vi "Editor Soglie pedrollo.vi"(11 "COLLEGAMENTO":u16(ring) items=["3-MOTORE C.A."]) -> ()   [LabVIEW 2019]
uses:
  TypeDef/DT TRASFORMATORE.ctl
  TypeDef/DT POMPA EXX.ctl
  TypeDef/DT POMPA.ctl
  TypeDef/DT MOTORE CC.ctl
  TypeDef/MOTORE EEX.ctl
  TypeDef/DT MOTORE CA.ctl
  TypeDef/DT GENERICO.ctl
  TypeDef/DT GENERATORE.ctl
  <vilib>/Utility/file.llb/Read Delimited Spreadsheet (string).vi
  <vilib>/Utility/file.llb/Write Delimited Spreadsheet (string).vi
panel:
  in  "Tab dati macchina":T1(tab)=enum."Page 4"
  in  "DATI MACCHINA-GENERATORE":T2
  in  "DATI MACCHINA-GENERICO":T3
  in  "DATI MACCHINA-MOTORE C.A.":T4
  in  "DATI MACCHINA-MOTORE EEX":T5
  in  "DATI MACCHINA-MOTORE C.C.":T6
  in  "DATI MACCHINA-POMPA":T7
  in  "DATI MACCHINA-POMPA EEX":T8
  in  "DATI MACCHINA-TRASFORMATORE":T9
  in  "salva soglie":bool
  in  "elimina soglia":bool
  in  "stop":bool
  in  "Cluster % NOMINALE":T10 {"VALORE NOMINALE BOLLETTINO" items=["3-MOTORE C.A.>>MARCA", "3-MOTORE C.A.>>TIPO", "3-MOTORE C.A.>>MATRICOLA", "3-MOTORE C.A.>>N°POLI", "3-MOTORE C.A.>>POTENZA [kW]", "3-MOTORE C.A.>>TENSIONE [V]", "3-MOTORE C.A.>>CORRENTE [A]", "3-MOTORE C.A.>>FREQUENZA [Hz]", "3-MOTORE C.A.>>RPM NOMINALI", "3-MOTORE C.A.>>RPM MAX", "3-MOTORE C.A.>>COSTRUTTORE", "3-MOTORE C.A.>>MODELLO Nr.", "3-MOTORE C.A.>>TIPO SERVIZIO", "3-MOTORE C.A.>>DESIGN", "3-MOTORE C.A.>>CLASSE ISOL", "3-MOTORE C.A.>>STATORE", "3-MOTORE C.A.>>ROTORE", "3-MOTORE C.A.>>NOTE"]; "RITARDO INTERVENTO" format="%#_g s"; "SOGLIA SUPERIORE" format="%#_g %"; "SOGLIA INFERIORE" format="%#_g %"}
  in  "SOGLIE INSERITE":i32(listbox)
  in  "Cluster COSTANTE":T11
  in  "costante \\ dinamica":bool=TRUE caption="SOGLIA COSTANTE\n\nSOGLIA DINAMICA\n% VALORE NOMINALE"
  in  "inserisci soglia":bool
  in  "Listbox":i32(listbox)
  # "GESTIONE SOGLIE"
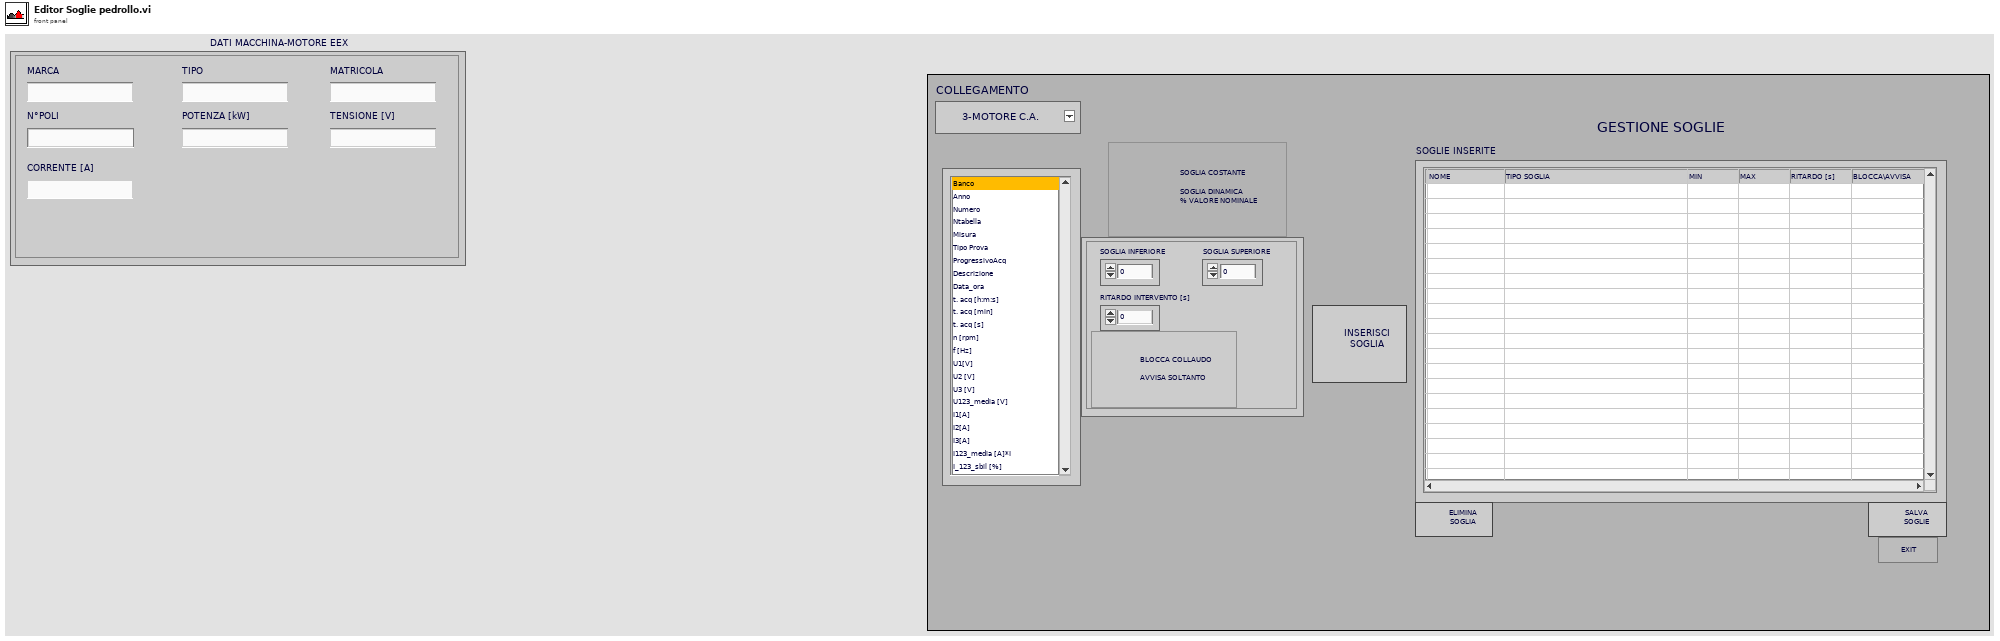
[diagram p1: front panel]
types:
  T1 = enum32{"Page 1", "Page 2", "Page 3", "Page 4", "Page 5", "Page 6", "Page 7", "Page 8"}
  T2 = typedef "DT GENERATORE.ctl" = cluster{"MARCA GENERATORE":string, "MARCA MOTORE":string, "MARCA ALTERNATORE":string, "MATRICOLA ALTERNATORE":string, "POTENZA [KVA]":string, "TENSIONE [V]":string, "CORRENTE [A]":string, "N° POLI":string, "GIRI [RPM]":string, "FREQUENZA [Hz]":string, "TENSIONE ECCIT.[V]":string, "CORRENTE ECCIT.[A]":string}
  T3 = typedef "DT GENERICO.ctl" = cluster{"MARCA":string, "TIPO":string, "MATRICOLA":string, "POTENZA [kW]":string, "TENSIONE [V]":string, "CORRENTE [A]":string}
  T4 = typedef "DT MOTORE CA.ctl" = cluster{"MARCA":string, "TIPO":string, "MATRICOLA":string, "N°POLI":string, "POTENZA [kW]":string, "TENSIONE [V]":string, "CORRENTE [A]":string, "FREQUENZA [Hz]":string, "RPM NOMINALI":string, "RPM MAX":string, "COSTRUTTORE":string, "MODELLO Nr.":string, "TIPO SERVIZIO":string, "DESIGN":string, "CLASSE ISOL":string, "STATORE":string, "ROTORE":string, "NOTE":string}
  T5 = typedef "MOTORE EEX.ctl" = cluster{"MARCA":string, "TIPO":string, "MATRICOLA":string, "N°POLI":string, "POTENZA [kW]":string, "TENSIONE [V]":string, "CORRENTE [A]":string}
  T6 = typedef "DT MOTORE CC.ctl" = cluster{"MARCA":string, "TIPO":string, "MATRICOLA":string, "POTENZA [kW]":string, "TENSIONE ARMAT.[V]":string, "CORRENTE ARMAT.[A]":string, "TENSIONE CAMPO [V]":string, "CORRENTE CAMPO [A]":string, "GIRI [RPM]":string, "TENSIONE DINAMO [V]":string}
  T7 = typedef "DT POMPA.ctl" = cluster{"MARCA":string, "TIPO":string, "MATRICOLA":string, "N°POLI":string, "POTENZA [kW]":string, "TENSIONE [V]":string, "CORRENTE [A]":string}
  T8 = typedef "DT POMPA EXX.ctl" = cluster{"MARCA":string, "TIPO":string, "MATRICOLA":string, "N°POLI":string, "POTENZA [kW]":string, "TENSIONE [V]":string, "CORRENTE [A]":string}
  T9 = typedef "DT TRASFORMATORE.ctl" = cluster{"MARCA":string, "TIPO":string, "MATRICOLA":string, "POTENZA [kW]":string, "TENSIONE PRIM. [V]":string, "CORRENTE PRIM. [A]":string, "TENSIONE SECON. [V]":string, "CORRENTE SECON. [A]":string, "GRUPPO CEI":string, "VCC%":string}
  T10 = cluster{"SOGLIA INFERIORE":dbl, "SOGLIA SUPERIORE":dbl, "RITARDO INTERVENTO":dbl, "blocca \\ avvisa":bool, "VALORE NOMINALE BOLLETTINO":u16}
  T11 = cluster{"SOGLIA INFERIORE":dbl, "SOGLIA SUPERIORE":dbl, "RITARDO INTERVENTO [s]":dbl, "blocca \\ avvisa":bool}
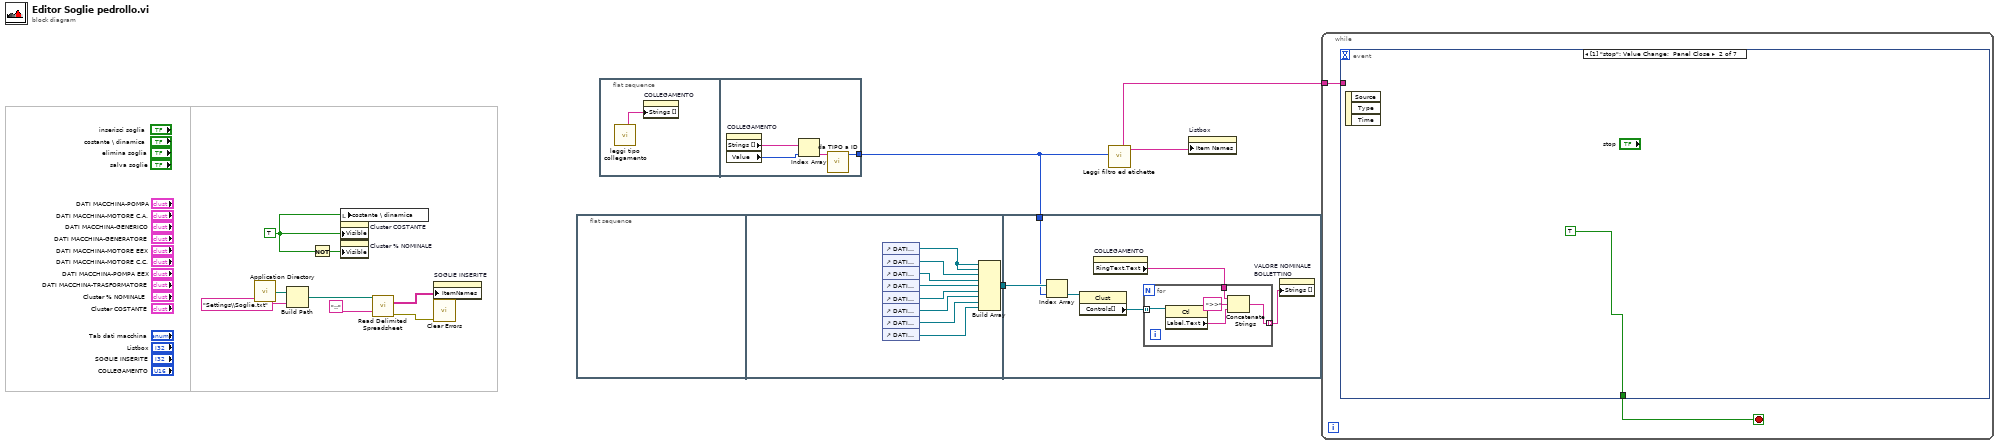
[diagram p0: block diagram]
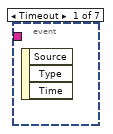
[diagram p2: hidden frame]
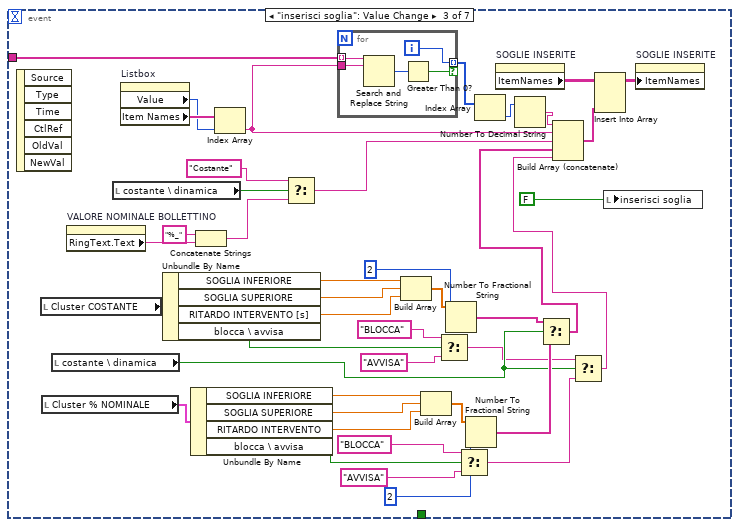
[diagram p3: hidden frame]
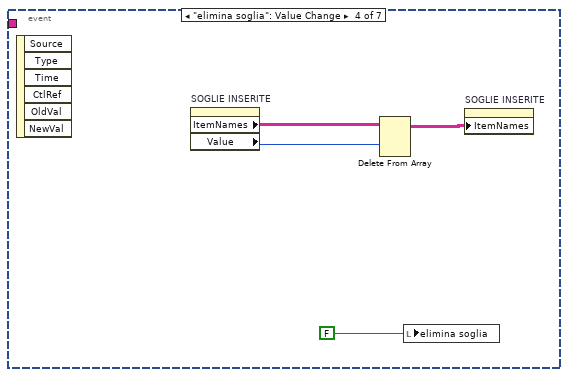
[diagram p4: hidden frame]
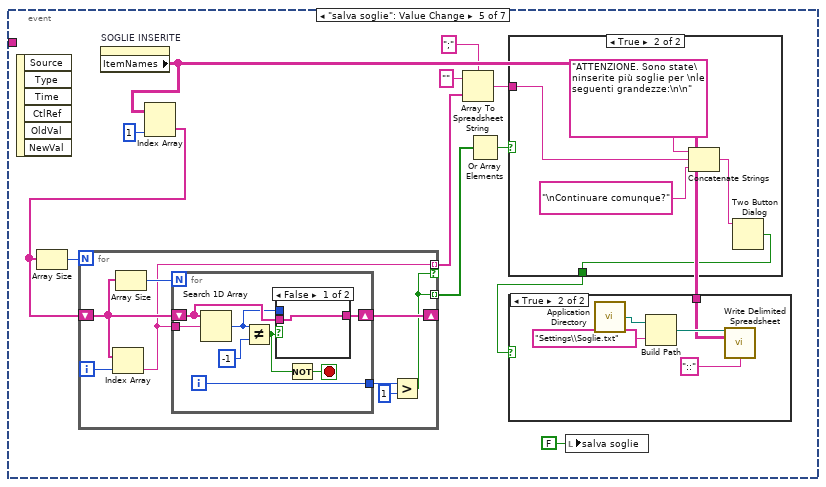
[diagram p5: hidden frame]
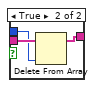
[diagram p6: hidden frame]
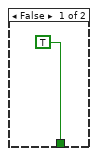
[diagram p8: hidden frame]
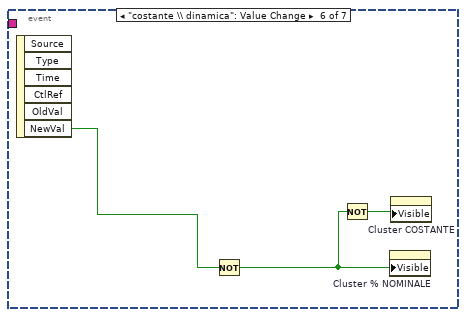
[diagram p9: hidden frame]
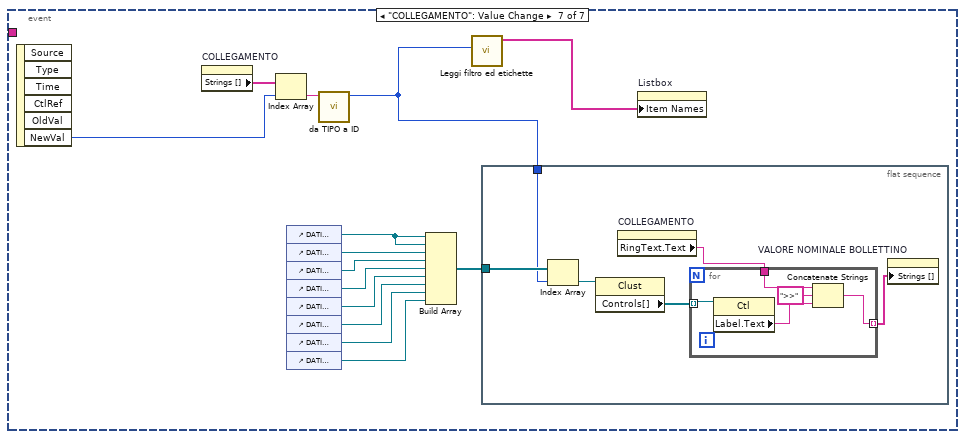
[diagram p10: hidden frame]
diagram:
  w6 = TRUE ("costante \\ dinamica")
  n1 = call <vilib>:"Application Directory.vi"() -> ("Application Directory"=w11:path)
  n2 = Build Path(base path=w11, name or relative path="Settings\\Soglie.txt") -> (appended path=w12:path)
  n3 = Not(x=w6) -> (.not. x?=w5:bool)
  n4 = local write "costante \\ dinamica"(w6) -> ()
  n5 = property on="Cluster COSTANTE" class="Clust (strict)"("Visible"=w6) -> ()  [unwired: 2 in, 2 out]
  n6 = property on="Cluster % NOMINALE" class="Clust (strict)"("Visible"=w5) -> ()  [unwired: 2 in, 2 out]
  n7 = call-poly <vilib>:"Read Delimited Spreadsheet.vi"("file path (dialog if empty)"=w12, "delimiter (\\t)"="::" ("delimiter (\\t)")) -> ("all rows"=w8:string[][], "error out"=w7:errorcluster)  [unwired: 8 in, 4 out]
  n8 = property on="SOGLIE INSERITE" class="MCListbox (strict)"("ItemNames"=w8) -> ()  [unwired: 2 in, 2 out]
  n9 = call <vilib>:"Clear Errors.vi"("error in (no error)"=w7) -> ()  [unwired: 5 in, 2 out]
  n10 = flat-sequence {
    tunnel: [w13] -> w1
    tunnel: w2 -> [w24]
    tunnel: w1 -> [w25]
    frame #0 {
    }
    frame #1 {
      n11 = control-ref of="DATI MACCHINA-GENERATORE"() -> (w14:refnum<vi>)
      n12 = control-ref of="DATI MACCHINA-GENERICO"() -> (w15:refnum<vi>)
      n13 = control-ref of="DATI MACCHINA-MOTORE C.A."() -> (w16:refnum<vi>)
      n14 = control-ref of="DATI MACCHINA-MOTORE EEX"() -> (w17:refnum<vi>)
      n15 = control-ref of="DATI MACCHINA-MOTORE C.C."() -> (w18:refnum<vi>)
      n16 = control-ref of="DATI MACCHINA-POMPA"() -> (w19:refnum<vi>)
      n17 = control-ref of="DATI MACCHINA-TRASFORMATORE"() -> (w20:refnum<vi>)
      n18 = control-ref of="DATI MACCHINA-POMPA EEX"() -> (w21:refnum<vi>)
      n19 = Build Array(w14, w14, w15, w16, w17, w18, w19, w20, w21) -> (w13:refnum<vi>[])
    }
    frame #2 {
      n20 = Index Array(array=w25, index=w24) -> (element=w23:refnum<vi>)
      n21 = property class="Clust"(reference=w23) -> ("Controls[]"=w26:refnum<vi>[])  [unwired: 1 in, 2 out]
      n22 = property on="COLLEGAMENTO" class="Ring (strict)"() -> ("RingText.Text"=w22:string)  [unwired: 2 in, 2 out]
      n23 = for {
        tunnel: w26 -> [w32] mode=indexing
        tunnel: [w30] -> w27 mode=indexing
        tunnel: w22 -> [w29]
        n24 = property class="Ctl"(reference=w32) -> ("Label.Text"=w31:string)  [unwired: 1 in, 2 out]
        n25 = Concatenate Strings(w29, ">>" ("string"), w31) -> (w30:string)
      }
      n26 = property on="VALORE NOMINALE BOLLETTINO" class="Ring (strict)"("Strings []"=w27) -> ()  [unwired: 2 in, 2 out]
    }
  }
  n27 = flat-sequence {
    tunnel: [w34] -> w2
    frame #0 {
      n28 = call "leggi tipo collegamento.vi"() -> ("lista"=w33:string[])  [unwired: 6 in, 5 out]
      n29 = property on="COLLEGAMENTO" class="Ring (strict)"("Strings []"=w33) -> ()  [unwired: 2 in, 2 out]
    }
    frame #1 {
      n30 = property on="COLLEGAMENTO" class="Ring (strict)"() -> ("Strings []"=w37:string[], "Value"=w36:u16)  [unwired: 2 in, 2 out]
      n31 = Index Array(array=w37, index=w36) -> (element=w35:string)
      n32 = call "da TIPO a ID.vi"("TIPO"=w35) -> ("ID"=w34:i32)  [unwired: 10 in]
    }
  }
  n33 = call "Leggi filtro ed etichette.vi"("ID COLLEGAMENTO"=w2) -> ("ETICHETTE"=w3:string[], "ALL"=w4:string[])  [unwired: 5 in, 4 out]
  n34 = property on="Listbox" class="LstBox (strict)"("Item Names"=w3) -> ()  [unwired: 2 in, 2 out]
  n35 = while {
    tunnel: w4 -> [w38]
    stop <- w39 stop-if-true
    n36 = event shown="[1] \"stop\": Value Change;  Panel Close" {
      selector: _ -> [_ _ _ _ _ _ _]
      dyn-events: _ -> [_ _ _ _ _ _ _]
      timeout: _ -> [_ _ _ _ _ _ _]
      tunnel: [_ TRUE _ _ _ _ _] -> w39
      tunnel: w38 -> [_ _ w47 _ _ _ _]
      event Timeout {
        n37 = event-data() -> ()  [unwired: 1 in, 3 out]
      }
      event "stop": Value Change; Panel Close {
        n38 = event-data() -> ()  [unwired: 1 in, 3 out]
      }
      event "inserisci soglia": Value Change {
        n39 = event-data() -> ()  [unwired: 1 in, 6 out]
        n40 = local read "Cluster COSTANTE"() -> (w68:T11)
        n41 = local read "Cluster % NOMINALE"() -> (w60:T10)
        n42 = local read "costante \\ dinamica"() -> (w56:bool)
        n43 = property on="VALORE NOMINALE BOLLETTINO" class="Ring (strict)"() -> ("RingText.Text"=w78:string)  [unwired: 2 in, 2 out]
        n44 = local read "costante \\ dinamica"() -> (w80:bool)
        n45 = property on="Listbox" class="LstBox (strict)"() -> ("Value"=w81:i32, "Item Names"=w82:string[])  [unwired: 2 in, 2 out]
        n46 = Unbundle By Name(w68) -> ("SOGLIA INFERIORE"=w72:dbl, "SOGLIA SUPERIORE"=w71:dbl, "RITARDO INTERVENTO [s]"=w70:dbl, "blocca \\ avvisa"=w75:bool)
        n47 = Unbundle By Name(w60) -> ("SOGLIA INFERIORE"=w64:dbl, "SOGLIA SUPERIORE"=w65:dbl, "RITARDO INTERVENTO"=w66:dbl, "blocca \\ avvisa"=w61:bool)
        n48 = Concatenate Strings("%_" ("string"), w78) -> (w76:string)
        n49 = Index Array(array=w82, index=w81) -> (element=w46:string)
        n50 = Select(t="Costante", s=w80, f=w76) -> (s? t:f=w41:string)
        n51 = for {
          tunnel: w47 -> [w87] mode=indexing
          tunnel: w46 -> [w86]
          tunnel: [w85] -> w45 mode=indexing if=w83
          i -> [w85]
          n52 = Search and Replace String(input string=w87, search string=w86) -> (number of replacements=w84:i32)  [unwired: 6 in, 3 out]
          n53 = Greater Than 0?(x=w84) -> (x > 0?=w83:bool)
        }
        n54 = Build Array(w72, w71, w70) -> (w69:dbl[])
        n55 = Build Array(w64, w65, w66) -> (w67:dbl[])
        n56 = Select(t="BLOCCA", s=w75, f="AVVISA") -> (s? t:f=w55:string)
        n57 = Number To Fractional String(number=w69, precision (6)=i16 2) -> (F-format string=w59:string[])  [unwired: 2 in]
        n58 = Select(t="BLOCCA", s=w61, f="AVVISA") -> (s? t:f=w54:string)
        n59 = Number To Fractional String(number=w67, precision (6)=i16 2) -> (F-format string=w58:string[])  [unwired: 2 in]
        n60 = Index Array(array=w45) -> (element=w44:i32)  [unwired: 1 in]
        n61 = property on="SOGLIE INSERITE" class="MCListbox (strict)"() -> ("ItemNames"=w52:string[][])  [unwired: 2 in, 2 out]
        n62 = Number To Decimal String(number=w44) -> (decimal integer string=w43:string)  [unwired: 1 in]
        n63 = Select(t=w59, s=w56, f=w58) -> (s? t:f=w57:string[])
        n64 = Select(t=w55, s=w56, f=w54) -> (s? t:f=w53:string)
        n65 = Build Array (concatenate)(w43, w46, w41, w57, w53) -> (w50:string[])
        n66 = Insert Into Array(array=w52, new element=w50) -> (w51:string[][])  [unwired: 2 in]
        n67 = local write "inserisci soglia"(FALSE ("inserisci soglia")) -> ()
        n68 = property on="SOGLIE INSERITE" class="MCListbox (strict)"("ItemNames"=w51) -> ()  [unwired: 2 in, 2 out]
      }
      event "elimina soglia": Value Change {
        n69 = event-data() -> ()  [unwired: 1 in, 6 out]
        n70 = property on="SOGLIE INSERITE" class="MCListbox (strict)"() -> ("ItemNames"=w91:string[][], "Value"=w90:i32)  [unwired: 2 in, 2 out]
        n71 = Delete From Array(array=w91, index (row)=w90) -> (array with subset deleted=w89:string[][])  [unwired: 2 in, 1 out]
        n72 = local write "elimina soglia"(FALSE ("elimina soglia")) -> ()
        n73 = property on="SOGLIE INSERITE" class="MCListbox (strict)"("ItemNames"=w89) -> ()  [unwired: 2 in, 2 out]
      }
      event "salva soglie": Value Change {
        n74 = event-data() -> ()  [unwired: 1 in, 6 out]
        n75 = property on="SOGLIE INSERITE" class="MCListbox (strict)"() -> ("ItemNames"=w102:string[][])  [unwired: 2 in, 2 out]
        n76 = Index Array(array=w102, index (col)=1 ("disabled index (col)")) -> (element=w94:string[])  [unwired: 1 in]
        n77 = Array Size(array=w94) -> (size(s)=w95:i32)
        n78 = for {
          N: w95 -> [_]
          tunnel: [w108] -> w93 mode=indexing if=w104
          shift-right: [w107] -> _
          shift-left: w94 -> [w110]
          tunnel: [w104] -> w92 mode=indexing
          i -> [w109]
          n79 = Index Array(array=w110, index=w109) -> (element=w108:string)
          n80 = Array Size(array=w110) -> (size(s)=w111:i32)
          n81 = for {
            N: w111 -> [_]
            tunnel: w108 -> [w119]
            shift-right: [w116] -> w107
            shift-left: w110 -> [w117]
            tunnel: [w112] -> w106
            i -> [w112]
            stop <- w113 stop-if-true
            n82 = Search 1D Array(1D array=w117, element=w119) -> (index of element=w115:i32)  [unwired: 1 in]
            n83 = Not Equal?(x=w115, y=-1) -> (x != y?=w114:bool)
            n84 = case shown="False" w114 {
              tunnel: w117 -> [w120 w123]
              tunnel: [w120 w122] -> w116
              tunnel: w115 -> [_ w121]
              frame False {
              }
              frame True {
                n85 = Delete From Array(array=w123, index=w121) -> (array with subset deleted=w122:string[])  [unwired: 1 in, 1 out]
              }
            }
            n86 = Not(x=w114) -> (.not. x?=w113:bool)
          }
          n87 = Greater?(x=w106, y=1) -> (0:w104:bool)
        }
        n88 = Array To Spreadsheet String(delimiter (Tab)=";", array=w93, 3:"" ("format string")) -> (spreadsheet string=w96:string)
        n89 = Or Array Elements(Boolean array=w92) -> (logical OR=w98:bool)
        n90 = case shown="True" w98 {
          tunnel: [TRUE w134] -> w97
          tunnel: w96 -> [_ w132]
          frame False {
          }
          frame True {
            n91 = Concatenate Strings("ATTENZIONE. Sono state\ninserite più soglie per \nle seguenti grandezze:\n\n" ("message"), w132, "\nContinuare comunque?" ("string")) -> (w131:string)
            n92 = Two Button Dialog(message=w131) -> (T button?=w134:bool)  [unwired: 2 in]
          }
        }
        n93 = case shown="True" w97 {
          tunnel: w102 -> [_ w124]
          frame False {
          }
          frame True {
            n94 = call <vilib>:"Application Directory.vi"() -> ("Application Directory"=w126:path)
            n95 = Build Path(base path=w126, name or relative path="Settings\\Soglie.txt") -> (appended path=w125:path)
            n96 = call-poly <vilib>:"Write Delimited Spreadsheet.vi"("file path (dialog if empty)"=w125, "2D data"=w124, "delimiter (\\t)"="::" ("delimiter (\\t)")) -> ()  [unwired: 11 in, 2 out]
          }
        }
        n97 = local write "salva soglie"(FALSE ("salva soglie")) -> ()
      }
      event "costante \\ dinamica": Value Change {
        n98 = event-data() -> ("NewVal"=w137:bool)  [unwired: 1 in, 5 out]
        n99 = Not(x=w137) -> (.not. x?=w136:bool)
        n100 = Not(x=w136) -> (.not. x?=w135:bool)
        n101 = property on="Cluster % NOMINALE" class="Clust (strict)"("Visible"=w136) -> ()  [unwired: 2 in, 2 out]
        n102 = property on="Cluster COSTANTE" class="Clust (strict)"("Visible"=w135) -> ()  [unwired: 2 in, 2 out]
      }
      event "COLLEGAMENTO": Value Change {
        n103 = event-data() -> ("NewVal"=w138:u16)  [unwired: 1 in, 5 out]
        n104 = property on="COLLEGAMENTO" class="Ring (strict)"() -> ("Strings []"=w140:string[])  [unwired: 2 in, 2 out]
        n105 = Index Array(array=w140, index=w138) -> (element=w141:string)
        n106 = control-ref of="DATI MACCHINA-GENERATORE"() -> (w142:refnum<vi>)
        n107 = control-ref of="DATI MACCHINA-GENERICO"() -> (w143:refnum<vi>)
        n108 = control-ref of="DATI MACCHINA-MOTORE C.A."() -> (w144:refnum<vi>)
        n109 = control-ref of="DATI MACCHINA-MOTORE EEX"() -> (w145:refnum<vi>)
        n110 = control-ref of="DATI MACCHINA-MOTORE C.C."() -> (w146:refnum<vi>)
        n111 = control-ref of="DATI MACCHINA-POMPA"() -> (w147:refnum<vi>)
        n112 = control-ref of="DATI MACCHINA-TRASFORMATORE"() -> (w148:refnum<vi>)
        n113 = control-ref of="DATI MACCHINA-POMPA EEX"() -> (w149:refnum<vi>)
        n114 = call "da TIPO a ID.vi"("TIPO"=w141) -> ("ID"=w139:i32)  [unwired: 10 in]
        n115 = Build Array(w142, w142, w143, w144, w145, w146, w147, w148, w149) -> (w150:refnum<vi>[])
        n116 = call "Leggi filtro ed etichette.vi"("ID COLLEGAMENTO"=w139) -> ("ETICHETTE"=w151:string[])  [unwired: 5 in, 5 out]
        n117 = flat-sequence {
          tunnel: w139 -> [w154]
          tunnel: w150 -> [w155]
          frame #0 {
            n118 = Index Array(array=w155, index=w154) -> (element=w153:refnum<vi>)
            n119 = property class="Clust"(reference=w153) -> ("Controls[]"=w156:refnum<vi>[])  [unwired: 1 in, 2 out]
            n120 = property on="COLLEGAMENTO" class="Ring (strict)"() -> ("RingText.Text"=w152:string)  [unwired: 2 in, 2 out]
            n121 = for {
              tunnel: w156 -> [w162] mode=indexing
              tunnel: [w160] -> w157 mode=indexing
              tunnel: w152 -> [w159]
              n122 = property class="Ctl"(reference=w162) -> ("Label.Text"=w161:string)  [unwired: 1 in, 2 out]
              n123 = Concatenate Strings(w159, ">>" ("string"), w161) -> (w160:string)
            }
            n124 = property on="VALORE NOMINALE BOLLETTINO" class="Ring (strict)"("Strings []"=w157) -> ()  [unwired: 2 in, 2 out]
          }
        }
        n125 = property on="Listbox" class="LstBox (strict)"("Item Names"=w151) -> ()  [unwired: 2 in, 2 out]
      }
    }
  }
